vi "Initialize.vi"(0 "Tone in":refnum<class "Tone.lvclass">, 1 "Filter in":refnum<class "Filter.lvclass">, 5 "Level in":refnum<class "Level.lvclass">, 7 "Fs (Hz)":dbl, 9 "Npts":i32, 11 "error in (no error)":errorcluster, 13 "Channel Name":string) -> (3 "Filter out":refnum<class "Filter.lvclass">, 4 "Tone out":refnum<class "Tone.lvclass">, 6 "Level out":refnum<class "Level.lvclass">, 15 "error out":errorcluster)   [LabVIEW 2020, in "Tone.lvclass"]
uses:
  Tone.lvclass
  Level/Level.lvclass
  Filter/Filter.lvclass
  Tone.lvclass/Tone.ctl
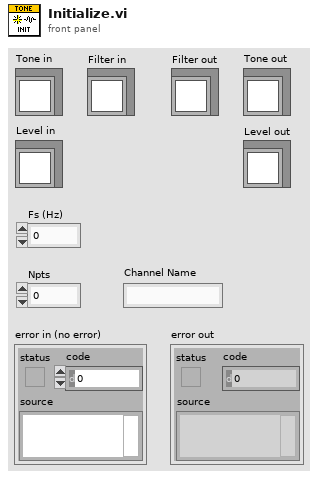
[diagram p1: front panel]
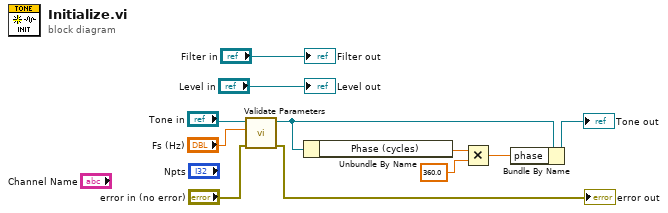
[diagram p0: block diagram]
diagram:
  n1 = call "Validate Parameters.vi"("error in (no error)"="error in (no error)", "Fs (Hz)"="Fs (Hz)", "Tone in"="Tone in") -> ("error out"=→"error out":errorcluster, "Tone out"=w7:refnum<class "Tone.lvclass">)  [unwired: 7 in]
  n2 = Unbundle By Name(w7) -> ("Phase (cycles)"=w5:dbl)
  n3 = Multiply(x=w5, y=360.0) -> (x*y=w3:dbl)
  n4 = Bundle By Name(cluster=w7, "phase"=w3) -> (→"Tone out":refnum<class "Tone.lvclass">)
  "Level out" <- "Level in"
  "Filter out" <- "Filter in"
